vi "magazine_state_machine.vi"(0 "Intake Button":bool, 1 "Outtake Button":bool, 2 "Both Sensors Active?":bool) -> (3 "Intake Pistons":bool, 4 "Magazine Motor":dbl, 5 "Intake Motor":dbl, 6 "Kicker Motor":dbl)   [LabVIEW 2020]
uses:
  magazine_state.ctl
panel:
  in  "Kicker Power":dbl=-1.0
  in  "Magazine Power":dbl=1.0
  in  "Intake Power":dbl=1.0
  # "Inputs"
  # "Power Levels"
  # "Outputs"
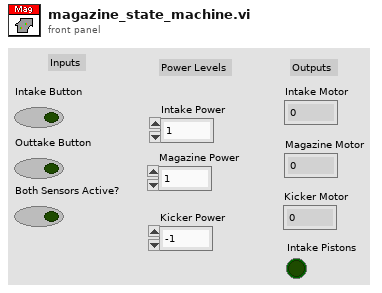
[diagram p1: front panel]
types:
  T1 = typedef "magazine_state.ctl" = enum16{"Idle", "Intake", "Outtake"}
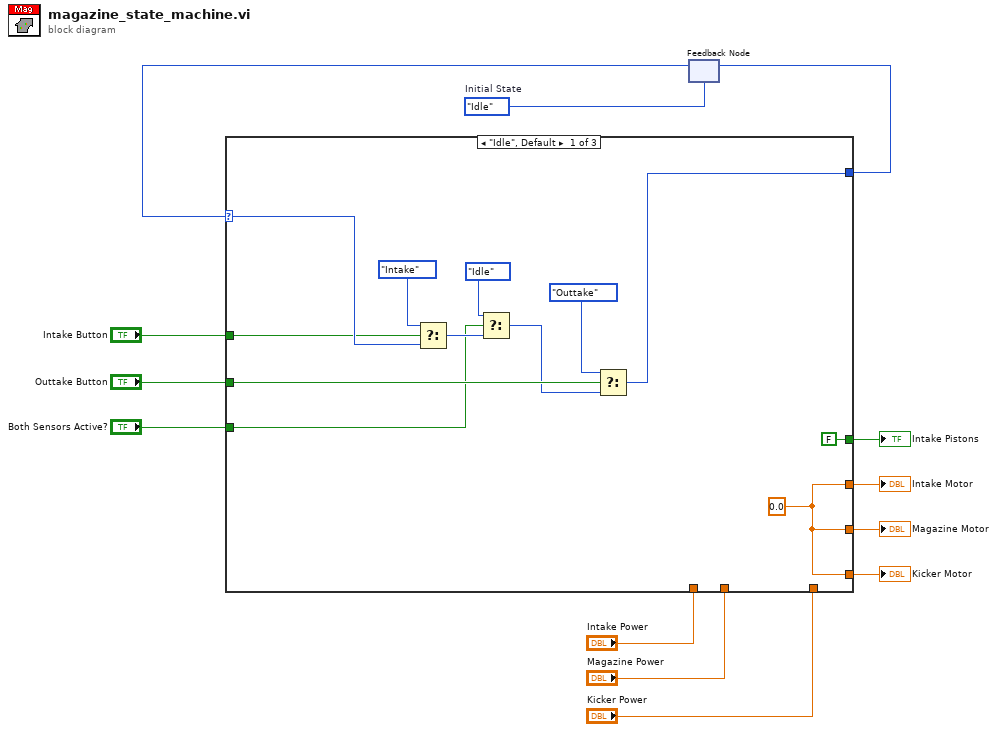
[diagram p0: block diagram]
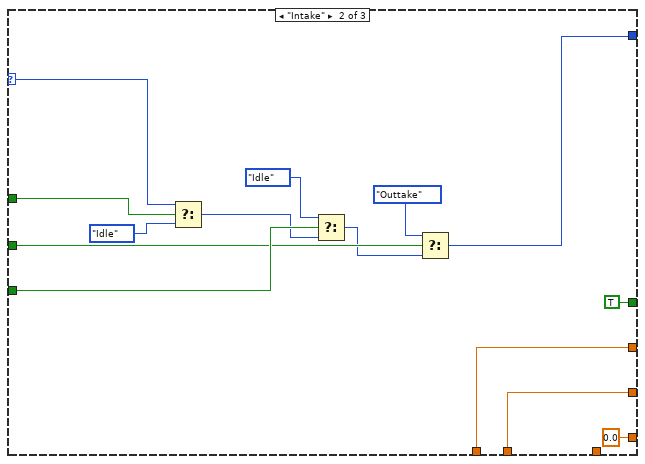
[diagram p2: hidden frame]
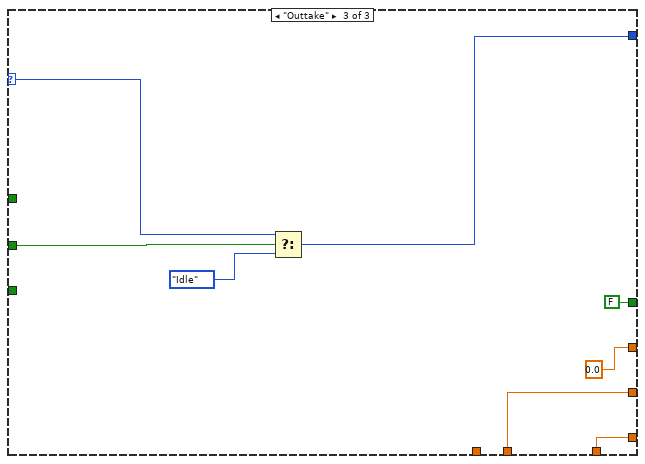
[diagram p3: hidden frame]
diagram:
  w2 = magazine_state."Idle"  # Initial State
  n1 = feedback #1(w2) -> (w4:T1)
  n2 = case shown="\"Idle\", Default" w4 {
    selector: w4 -> [w24 w38 w40]
    tunnel: "Intake Button" -> [w15 w39 _]
    tunnel: "Outtake Button" -> [w25 w28 w47]
    tunnel: "Both Sensors Active?" -> [w17 w36 _]
    tunnel: [w23 w33 0.0 ("Input Power")] -> w8
    tunnel: "Intake Power" -> [_ w33 _]
    tunnel: [w23 w32 w45] -> w10
    tunnel: "Magazine Power" -> [_ w32 w45]
    tunnel: [w23 0.0 ("Kicker Power") w42] -> w12
    tunnel: "Kicker Power" -> [_ _ w42]
    tunnel: [FALSE ("Intake Pistons") TRUE ("Intake Pistons") FALSE ("Intake Pistons")] -> w3
    tunnel: [w20 w26 w41] -> w1
    frame "Idle", Default {
      w23 = 0.0 ("Input Power")
      n3 = Select(t=magazine_state."Intake", s=w15, f=w24) -> (s? t:f=w19:T1)
      n4 = Select(t=magazine_state."Idle", s=w17, f=w19) -> (s? t:f=w16:T1)
      n5 = Select(t=magazine_state."Outtake", s=w25, f=w16) -> (s? t:f=w20:T1)
    }
    frame "Intake" {
      n6 = Select(t=w38, s=w39, f=magazine_state."Idle" ("t")) -> (s? t:f=w29:T1)
      n7 = Select(t=magazine_state."Idle", s=w36, f=w29) -> (s? t:f=w27:T1)
      n8 = Select(t=magazine_state."Outtake", s=w28, f=w27) -> (s? t:f=w26:T1)
    }
    frame "Outtake" {
      n9 = Select(t=w40, s=w47, f=magazine_state."Idle" ("t")) -> (s? t:f=w41:T1)
    }
  }
  "Intake Motor" <- w8
  "Magazine Motor" <- w10
  "Kicker Motor" <- w12
  "Intake Pistons" <- w3
  n10 = feedback-in #1(w1) -> ()
